vi "H5Lget_info.vi"(6 "lapl_id":T4, 8 "error in (no error)":errorcluster, 10 "Name":string, 11 "Location Ref":T4) -> (0 "error out":errorcluster, 2 "H5L_info_t":T1 {"cset" items=["H5T_CSET_ERROR"=-1, "H5T_CSET_ASCII"=0, "H5T_CSET_UTF8"=1]; "type" items=["H5L_TYPE_ERROR"=-1, "H5L_TYPE_HARD"=0, "H5L_TYPE_SOFT"=1, "H5L_TYPE_EXTERNAL"=64, "H5L_TYPE_MAX"=255]}, 3 "Location Ref out":T4)   [LabVIEW 2017]
doc: "Returns information about a link."
uses:
  <vilib>/UPVI/lvhdf5/library.llb/HDF5 Ref.ctl
  <vilib>/UPVI/lvhdf5/link.llb/H5L_info_t.ctl
  <vilib>/UPVI/lvhdf5/link.llb/H5L_type_t.ctl
  <vilib>/UPVI/lvhdf5/datatype.llb/H5T_cset_t.ctl
  <vilib>/UPVI/lvhdf5/hdf5.dll
  <vilib>/UPVI/lvhdf5/h5helper.dll
panel:
  # "LVHDF5 Toolkit\nCopyright (c) 2005-2013 by Jason D. Sommerville\nCopyright (c) 2014-2015 by UPVI, LLC.\n\nThis use and distribution of this file is governed by the terms found in \nLICENSE.txt distributed with this toolkit and installed at\n <user.lib>\\_lvhdf5\\LICENSE.txt"
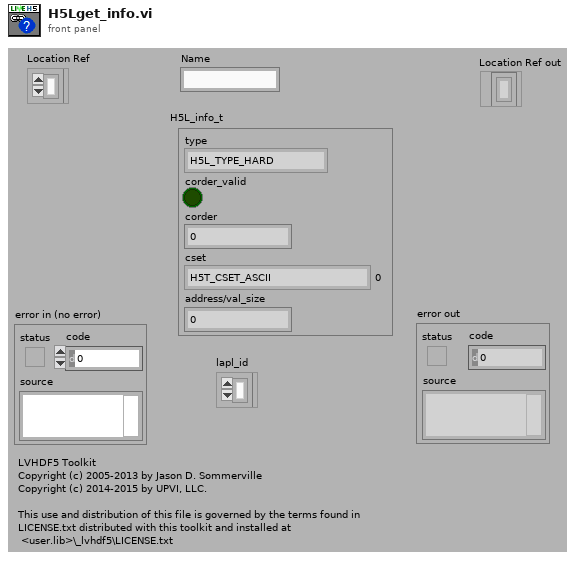
[diagram p1: front panel]
types:
  T1 = typedef "H5L_info_t.ctl" = cluster{"type":T2, "corder_valid":bool, "corder":i64, "cset":T3, "address/val_size":u64}
  T2 = typedef "H5L_type_t.ctl" = i32
  T3 = typedef "H5T_cset_t.ctl" = i32
  T4 = typedef "HDF5 Ref.ctl" = refnum<k1>
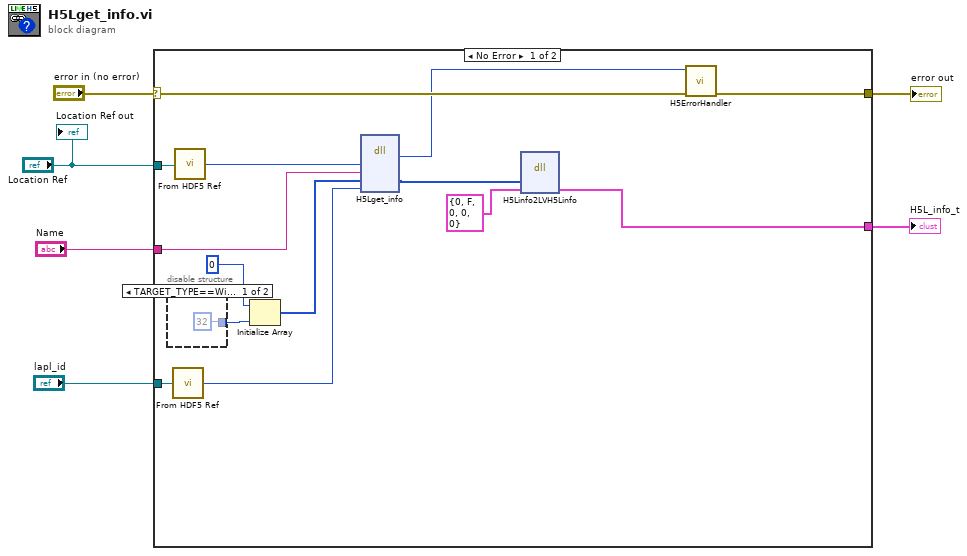
[diagram p0: block diagram]
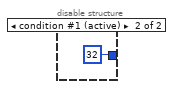
[diagram p2: hidden frame]
diagram:
  n1 = case shown="No Error" "error in (no error)" {
    selector: "error in (no error)" -> [w20 w23]
    tunnel: [w19 w23] -> w5
    tunnel: "lapl_id" -> [w18 _]
    tunnel: "Location Ref" -> [w15 _]
    tunnel: "Name" -> [w13 _]
    tunnel: [w7 _] -> w1
    frame No Error {
      n2 = disable-structure shown="TARGET_TYPE==Windows&&TARGET_BITNESS==32, default" {
        disable-tunnel: [32 32] -> w12
        frame condition #0 {
        }
        frame condition #1 (active) {
        }
      }
      n3 = call <vilib>:"From HDF5 Ref.vi"("HDF5 Ref"=w18) -> ("I32"=w17:i32)
      n4 = call <vilib>:"From HDF5 Ref.vi"("HDF5 Ref"=w15) -> ("I32"=w14:i32)
      n5 = Initialize Array(u8 0, w12) -> (w10:u8[])
      n6 = dll-call lib="C:/Program Files/National Instruments/LabVIEW 2017/vi.lib/UPVI/lvhdf5/hdf5.dll" fn="H5Lget_info"("dest_loc_id"=w14, "dest_name"=w13, "link_buff"=w10, "lapl_id"=w17) -> ("return type"=w16:i32, "link_buff"=w8:u8[])  [unwired: 6 in, 2 out]
      n7 = dll-call lib="C:/Program Files/National Instruments/LabVIEW 2017/vi.lib/UPVI/lvhdf5/h5helper.dll" fn="H5Linfo2LVH5Linfo"("H5Linfo"=w8, "LVH5Linfo"=T1 {"type"=0, "corder_valid"=FALSE, "corder"=0, "cset"=0, "address/val_size"=0} ("H5L_info_t")) -> ("LVH5Linfo"=w7:T1)  [unwired: 5 in, 2 out]
      n8 = call <vilib>:"H5ErrorHandler.vi"("error in (no error)"=w20, "herr_t"=w16) -> ("error out"=w19:errorcluster)  [unwired: 3 in, 4 out]
    }
    frame Error {
    }
  }
  "error out" <- w5
  "H5L_info_t" <- w1
  "Location Ref out" <- "Location Ref"
